vi "3A WriteToFIFOPort4.vi"(9 "String":string, 11 "Pre-existing reference":refnum<k20>) -> (2 "FPGA VI Reference Out":refnum<k20>)   [LabVIEW 2011]
doc: "Elizabeth Mahon and Olli Gallitz\n\nGiven an FPGA reference and input string, breaks the string into data to send down to the FPGA and from there the servo controller. Currently configured to work with Testbench for Servo.vi - the actual code should be fairly similar."
uses:
  <vilib>/FPGAPlugInAG/cRIO-9113/niLvFpga_Open_cRIO-9113.vi
  <vilib>/rvi/errors/niLvFpgaMergeErrorWithErrorCode.vi
  <vilib>/rvi/interface/nirviOpenFPGA/nirviOpenFPGA.xnode
  FPGA Bitfiles/SailBot_FPGATarget_3AFPGAReadFromFI_976E4797.lvbitx
  3A FPGA ReadFromFIFOPort4.vi
  <vilib>/rvi/interface/nirviMethod/nirviMethod.xnode
  <vilib>/FPGAPlugInAG/cRIO-9113/niLvFpga_WriteFifo_cRIO-9113.vi
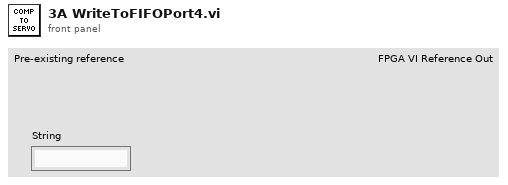
[diagram p1: front panel]
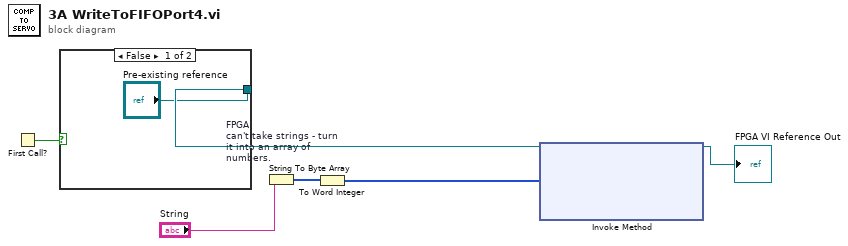
[diagram p0: block diagram]
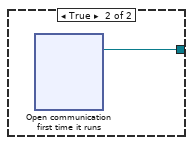
[diagram p2: hidden frame]
diagram:
  n1 = First Call?() -> (First Call?: T/F=w5:bool)
  n2 = case shown="False" w5 {
    tunnel: ["Pre-existing reference" w8] -> w4
    frame False {
    }
    frame True {
      n3 = xnode "Open communication\nfirst time it runs"() -> ("FPGA VI Reference Out"=w8:refnum<k20>)  [unwired: 2 in, 1 out]
    }
  }
  n4 = String To Byte Array "FPGA\ncan't take strings - turn it into an array of numbers."(string="String") -> (unsigned byte array=w2:u8[])
  n5 = To Word Integer(number=w2) -> (16bit integer=w1:i16[])
  n6 = xnode "Invoke Method"("FPGA VI Reference In"=w4, "Data"=w1) -> ("FPGA VI Reference Out"=→"FPGA VI Reference Out":refnum<k20>)  [unwired: 2 in, 2 out]
